vi "Clear Task.vi"(8 "error in":errorcluster, 11 "NI Waveform Output in":refnum<class "NI Waveform Output.lvclass">) -> (0 "error out":errorcluster, 3 "NI Waveform Output out":refnum<class "NI Waveform Output.lvclass">)   [LabVIEW 2023, in "HardwareAbstractionLayer_LVOOP.lvlib" / "NI Waveform Output.lvclass"]
doc: "DAQ AO Clear Data"
uses:
  NI Waveform Output.lvclass
  NI Waveform Output.lvclass/NI Waveform Output.ctl
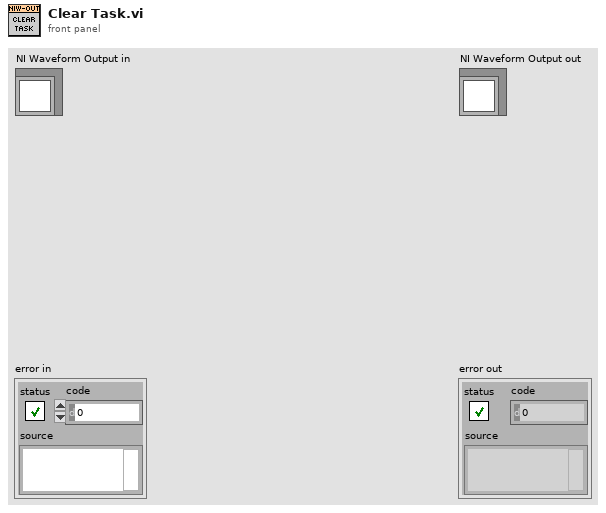
[diagram p1: front panel]
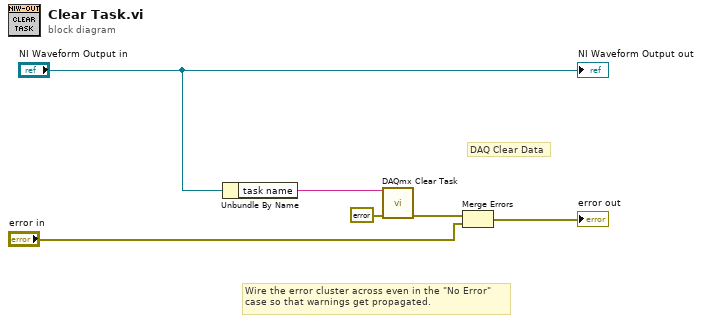
[diagram p0: block diagram]
diagram:
  # "DAQ Clear Data"
  # "Wire the error cluster across even in the \"No Error\"\ncase so that warnings get propagated."
  n1 = Unbundle By Name("NI Waveform Output in") -> ("task name"=w4:string)
  n2 = call <vilib>:"DAQmx Clear Task.vi"("task in"=w4, "error in"=errorcluster {"status"=FALSE, "code"=0, "source"=""}) -> ("error out"=w6:errorcluster)  [unwired: 13 in]
  n3 = Merge Errors(w6, "error in") -> (→"error out":errorcluster)
  "NI Waveform Output out" <- "NI Waveform Output in"
